vi "Initialise GUI.vi"(4 "View Buttons":refnum<vi>, 8 "error in (no error)":errorcluster, 11 "Main Controller in":refnum<class "Main Controller Actor.lvclass">) -> (0 "error out":errorcluster, 3 "Main Controller out":refnum<class "Main Controller Actor.lvclass">)   [LabVIEW 2021, in "Main Controller Actor.lvclass"]
uses:
  Main Controller Actor.lvclass
  Main Controller Actor.lvclass/Main Controller Actor.ctl
  Main INI/Main INI.lvlib
  Windows.ctl
  View.ctl
  Resource Manager/Resource Manager.lvclass
  Renderer/Renderer.lvclass
  Sprite Font/Sprite Font.lvclass
  Sprite Font/Game Font.ctl
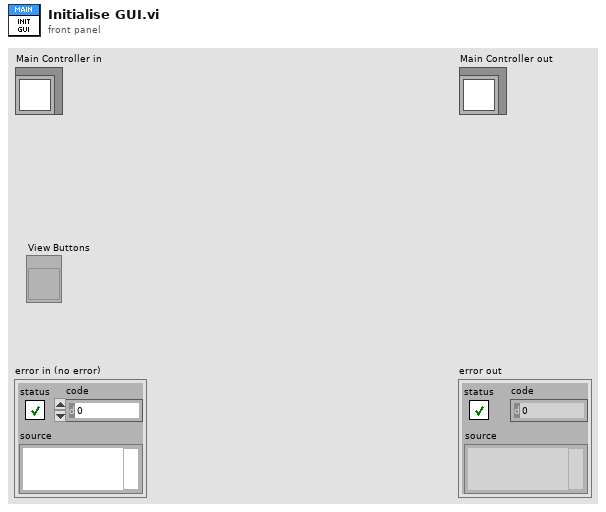
[diagram p1: front panel]
types:
  T1 = typedef "Sprite Font.lvclass/Game Font.ctl" = enum16{"Ilwrath", "Micro", "Slylandro", "Starcon", "Tiny", "Utwig"}
  T2 = typedef "Main Controller Actor.lvclass/View.ctl" = enum32{"Main", "Boolean", "Info", "Dev"}
  T3 = typedef "Main INI.lvlib/Core Data.ctl" = cluster{"Config":cluster{"System Config Name":string, "Debug":bool}}
  T4 = typedef "Main Controller Actor.lvclass/Windows.ctl" = enum16{"Debugger"}
  T5 = typedef "Constants.ctl" = cluster{"Colours":cluster{"OK":u32, "Warning":u32, "Error":u32, "Red":u32, "Green":u32, "Blue":u32, "Yellow":u32}, "System":cluster{"Target Frames Second":dbl, "World Size":T6, "Window Size":T6, "Battle Area Size":T6, "Sidebar Scaling":sgl, "Sidebar Width":i32, "SC2 Frame Rate [Seconds/Frame]":sgl}, "Game":cluster{"Maximum Asteroids":i32, "Max Energy":i32, "Max Crew":i32, "Maximum Stars":i32}}
  T6 = typedef "SDL2 Utility.lvlib/Point (I32).ctl" = cluster{"x":i32, "y":i32}
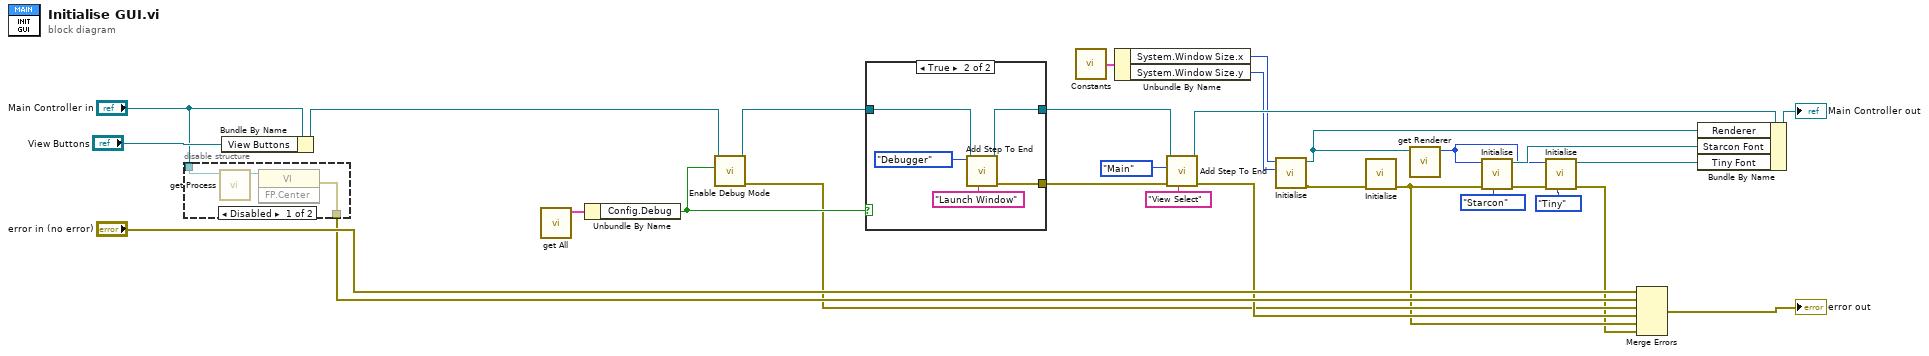
[diagram p0: block diagram]
diagram:
  n1 = disable-structure shown="Disabled" {
    disable-tunnel: [w32 _] -> w28
    disable-tunnel: "Main Controller in" -> [w31 _]
    frame Disabled {
      n2 = call-dynamic "get Process.vi"("Actor in"=w31) -> ("Process"=w33:refnum<vi>)  [unwired: 9 in, 1 out]
      n3 = invoke class="VI" method="FP.Center"(reference=w33) -> (error out=w32:errorcluster)  [unwired: 2 in, 2 out]
    }
    frame Enabled {
    }
  }
  n4 = Bundle By Name(cluster="Main Controller in", "View Buttons"="View Buttons") -> (w20:refnum<class "Main Controller Actor.lvclass">)
  n5 = call "get All.vi"() -> ("Data out"=w27:T3)  [unwired: 10 in, 1 out]
  n6 = Unbundle By Name(w27) -> ("Config.Debug"=w22:bool)
  n7 = call "Enable Debug Mode.vi"("Enable Debug"=w22, "Actor in"=w20) -> ("error out"=w17:errorcluster, "Actor out"=w16:refnum<class "Main Controller Actor.lvclass">)  [unwired: 8 in]
  n8 = case shown="True" w22 {
    tunnel: w16 -> [w34 w38]
    tunnel: [w34 w37] -> w25
    tunnel: [_ w35] -> w19
    frame False {
    }
    frame True {
      n9 = call-dynamic "Add Step To End.vi"("Step Name"="Launch Window", "Parameter"=Windows."Debugger" ("Window"), "Actor in"=w38) -> ("error out"=w35:errorcluster, "Actor out"=w37:refnum<class "Main Controller Actor.lvclass">)  [unwired: 7 in]
    }
  }
  n10 = call "Constants.vi"() -> ("Constants"=w12:T5)
  n11 = Unbundle By Name(w12) -> ("System.Window Size.x"=w11:i32, "System.Window Size.y"=w10:i32)
  n12 = call-dynamic "Add Step To End.vi"("Step Name"="View Select", "error in (no error)"=w19, "Parameter"=View."Main" ("View"), "Actor in"=w25) -> ("error out"=w18:errorcluster, "Actor out"=w14:refnum<class "Main Controller Actor.lvclass">)  [unwired: 6 in]
  n13 = call "Initialise.vi"("Window Height"=w10, "Window Width"=w11) -> ("error out"=w15:errorcluster, "Renderer out"=w8:refnum<class "Renderer.lvclass">)  [unwired: 8 in]
  n14 = call "Initialise.vi"("error in (no error)"=w15) -> ("error out"=w9:errorcluster)  [unwired: 10 in]
  n15 = call-dynamic "get Renderer.vi"("Renderer in"=w8) -> ("Renderer"=w5:u32)  [unwired: 10 in]
  n16 = call "Initialise.vi"("Font"=Game_Font."Starcon", "error in (no error)"=w9, "Renderer"=w5) -> ("error out"=w6:errorcluster, "Font out"=w7:refnum<class "Sprite Font.lvclass">)  [unwired: 7 in]
  n17 = call "Initialise.vi"("Font"=Game_Font."Tiny", "error in (no error)"=w6, "Renderer"=w5) -> ("error out"=w1:errorcluster, "Font out"=w2:refnum<class "Sprite Font.lvclass">)  [unwired: 7 in]
  n18 = Merge Errors("error in (no error)", w28, w17, w18, w9, w1) -> (→"error out":errorcluster)
  n19 = Bundle By Name(cluster=w14, "Renderer"=w8, "Starcon Font"=w7, "Tiny Font"=w2) -> (→"Main Controller out":refnum<class "Main Controller Actor.lvclass">)
